vi "Initialize.vi"(8 "error in (no error)":errorcluster, 10 "RESTLoader":refnum<class "RESTLoaderBase.lvclass">, 11 "REST in":refnum<class "RESTBase.lvclass">) -> (0 "error out":errorcluster, 3 "REST out":refnum<class "RESTBase.lvclass">)   [LabVIEW 2019, in "ByteREST.lvlib" / "RESTBase.lvclass"]
doc: "Apre una nuova connessione HTTP e setta il content type a \"application/json\""
uses:
  RESTBase.lvclass
  CfgLoaders/LoaderBase/RESTLoaderBase.lvclass
  RESTBase.lvclass/RESTBase.ctl
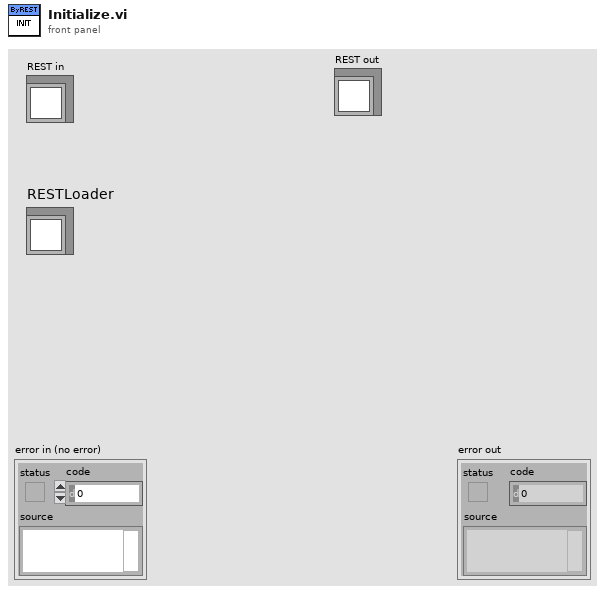
[diagram p1: front panel]
types:
  T1 = typedef "ByteREST.lvlib/RESTLoaderBase.lvclass/ServerParams.ctl" = cluster{"API Root":string, "verify server":bool, "Version (no version)":string, "Port (protocol specific)":u16, "Base URL":string, "Auth type":T2, "Auth string":string, "timeout (10000)":i32, "Token preamble (Token)":string, "Token empty preamble (False)":bool, "Token header key (Authorization)":string}
  T2 = typedef "ByteREST.lvlib/RESTBase.lvclass/Authentication_type.ctl" = enum16{"Token"}
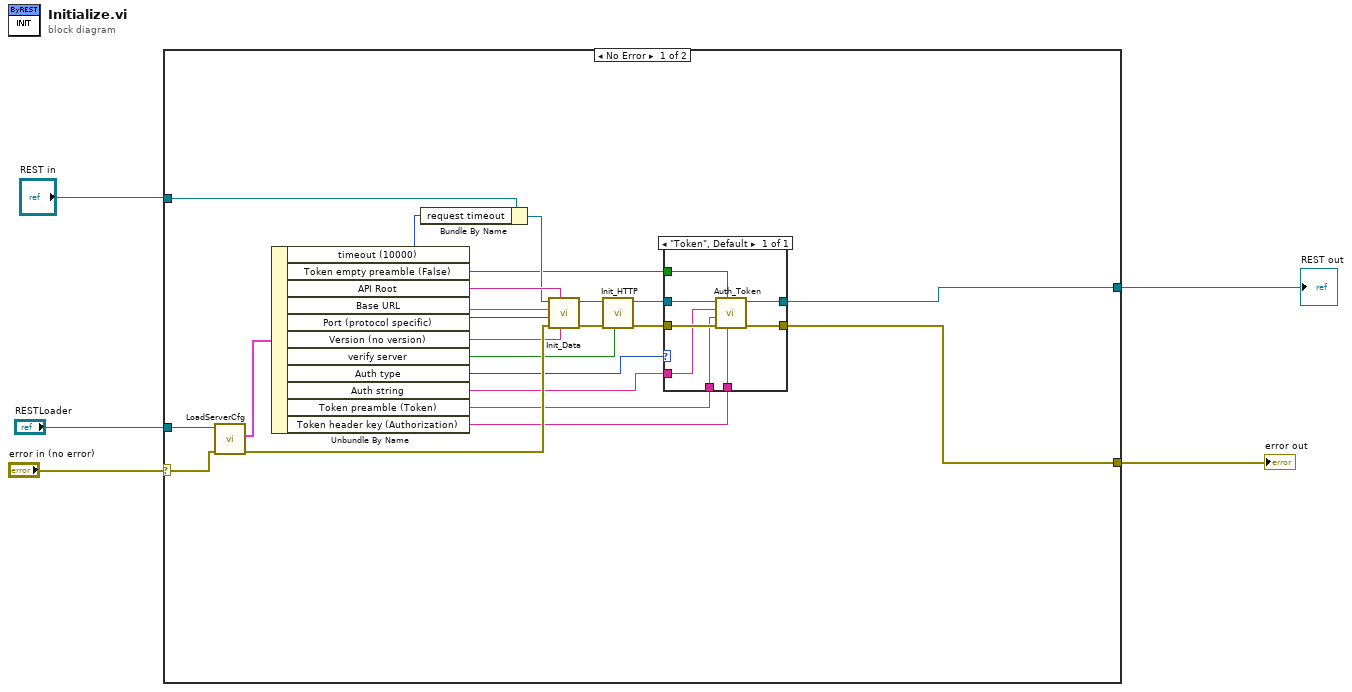
[diagram p0: block diagram]
diagram:
  n1 = case shown="No Error" "error in (no error)" {
    selector: "error in (no error)" -> [w20 w38]
    tunnel: [w23 w38] -> w4
    tunnel: [w22 w37] -> w2
    tunnel: "REST in" -> [w26 w37]
    tunnel: "RESTLoader" -> [w21 _]
    frame No Error {
      n2 = call-dynamic "LoadServerCfg.vi"("error in (no error)"=w20, "RESTLoaderBase in"=w21) -> ("error out"=w19:errorcluster, "Server config"=w18:T1)  [unwired: 7 in, 1 out]
      n3 = Unbundle By Name(w18) -> ("timeout (10000)"=w9:i32, "Token empty preamble (False)"=w6:bool, "API Root"=w17:string, "Base URL"=w16:string, "Port (protocol specific)"=w15:u16, "Version (no version)"=w14:string, "verify server"=w13:bool, "Auth type"=w12:T2, "Auth string"=w11:string, "Token preamble (Token)"=w8:string, "Token header key (Authorization)"=w7:string)
      n4 = Bundle By Name(cluster=w26, "request timeout"=w9) -> (w10:refnum<class "RESTBase.lvclass">)
      n5 = call "Init_Data.vi"("Version (no version)"=w14, "API Root"=w17, "error in (no error)"=w19, "Port (protocol specific)"=w15, "Base URL"=w16, "ByteGSAPIBase in"=w10) -> ("error out"=w27:errorcluster, "ByteGSAPIBase out"=w28:refnum<class "RESTBase.lvclass">)  [unwired: 4 in]
      n6 = call "Init_HTTP.vi"("verify server(true)"=w13, "error in (no error)"=w27, "ByteRESTBase in"=w28) -> ("error out"=w24:errorcluster, "ByteRESTBase out"=w25:refnum<class "RESTBase.lvclass">)  [unwired: 7 in]
      n7 = case shown="\"Token\", Default" w12 {
        tunnel: w25 -> [w36]
        tunnel: w24 -> [w35]
        tunnel: [w34] -> w23
        tunnel: [w33] -> w22
        tunnel: w11 -> [w32]
        tunnel: w8 -> [w31]
        tunnel: w7 -> [w30]
        tunnel: w6 -> [w29]
        frame "Token", Default {
          n8 = call "Auth_Token.vi"("Token header key (Authorization)"=w30, "Token empty preamble (False)"=w29, "error in (no error)"=w35, "Token preamble (Token)"=w31, "Token"=w32, "ByteGSAPIBase in"=w36) -> ("error out"=w34:errorcluster, "ByteGSAPIBase out"=w33:refnum<class "RESTBase.lvclass">)  [unwired: 4 in]
        }
      }
    }
    frame Error {
    }
  }
  "error out" <- w4
  "REST out" <- w2
